vi "ATDome_issueCommand_moveShutterMainDoor.vi"(8 "error in (no error)":errorcluster, 11 "command_moveShutterMainDoor_Ctl":T1) -> (0 "error out":errorcluster, 2 "function return":i32, 3 "command_moveShutterMainDoor_Ctl out":T1)   [LabVIEW 2016, in "SALLV_ATDome.lvlib"]
doc: "int ATDome_shm_issueCommand_moveShutterMainDoorLV(ATDome_command_moveShutterMainDoorLV *command_moveShutterMainDoor_Ctl );"
uses:
  SALLV_ATDome.lvlib
  DataTypes/command_moveShutterMainDoor.ctl
  SALLV_ATDome.so
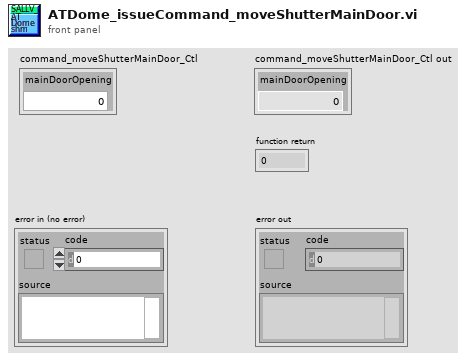
[diagram p1: front panel]
types:
  T1 = typedef "SALLV_ATDome.lvlib/command_moveShutterMainDoor.ctl" = cluster{"mainDoorOpening":sgl}
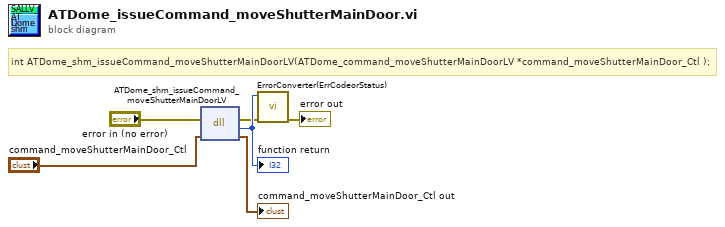
[diagram p0: block diagram]
diagram:
  # "int ATDome_shm_issueCommand_moveShutterMainDoorLV(ATDome_command_moveShutterMainDoorLV *command_moveShutterMainDoor_Ctl );"
  n1 = dll-call lib="home/andres/Desktop/SAL_ATDome/SALLV_ATDome.*" fn="ATDome_shm_issueCommand_moveShutterMainDoorLV"(error in="error in (no error)", "command_moveShutterMainDoor_Ctl"="command_moveShutterMainDoor_Ctl") -> (error out=w2:errorcluster, w6:i32, "command_moveShutterMainDoor_Ctl"=→"command_moveShutterMainDoor_Ctl out":T1)  [unwired: 2 in, 1 out]
  "function return" <- w6
  n2 = call "ErrorConverter(ErrCodeorStatus).vi"("error in (no error)"=w2, "error code"=w6) -> ("error out"=→"error out":errorcluster)  [unwired: 9 in]
